vi "TruPlasma3001.vi"() -> ()   [LabVIEW 2015]
panel:
  in  "Pset":dbl=150.0
  in  "Iset":dbl=5000.0
  in  "Uset":dbl=800.0
  in  "Byte string":string
  out "Bytes recieved":u32
  out "Bytes sent":u32
  in  "Boolean":bool
  out "string":string
  in  "CMD_L":string="ÿ"
  in  "CMD_H":string="ÿ"
  in  "reference":refnum<visa-resource-name>
  out "error out":errorcluster
  out "Command recieved":string
  # "Mains Relays: (1)On (0)Off\nPower: Off(0), On(1)\nReset arc counters: 1\n-\nAnalog: (1)\nPC Controls TruPlasma(1), Monitoring only(0)\nProfibus control(1)\nDisplay control(1)"
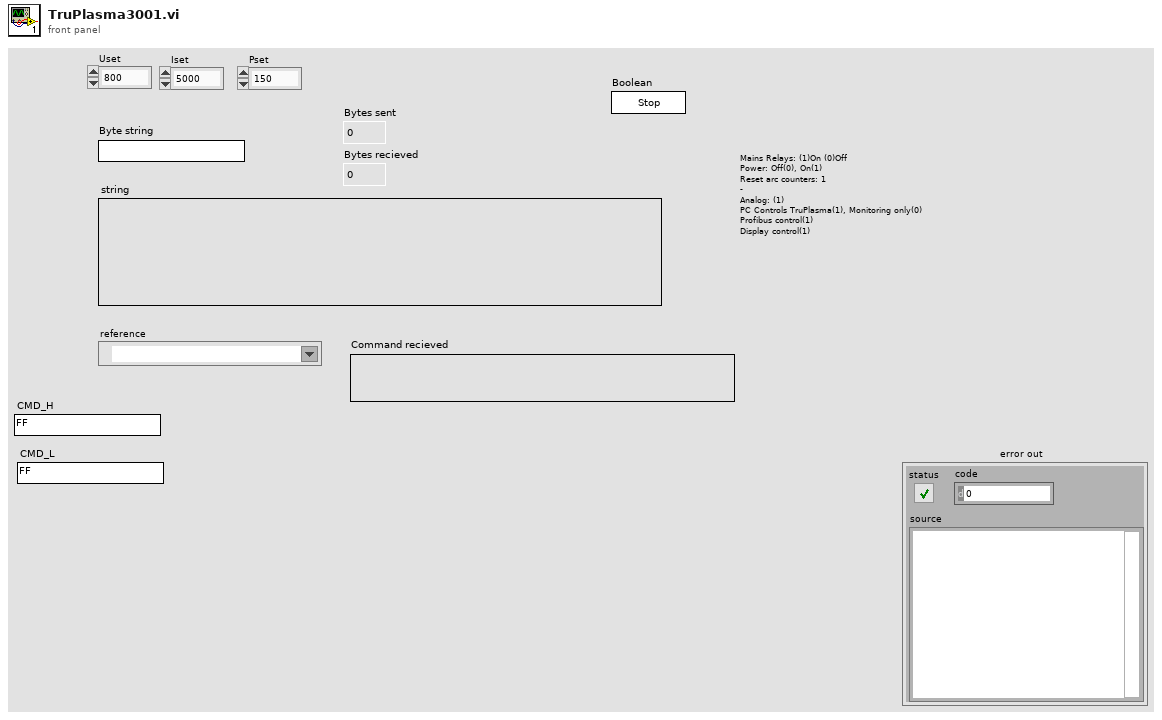
[diagram p1: front panel]
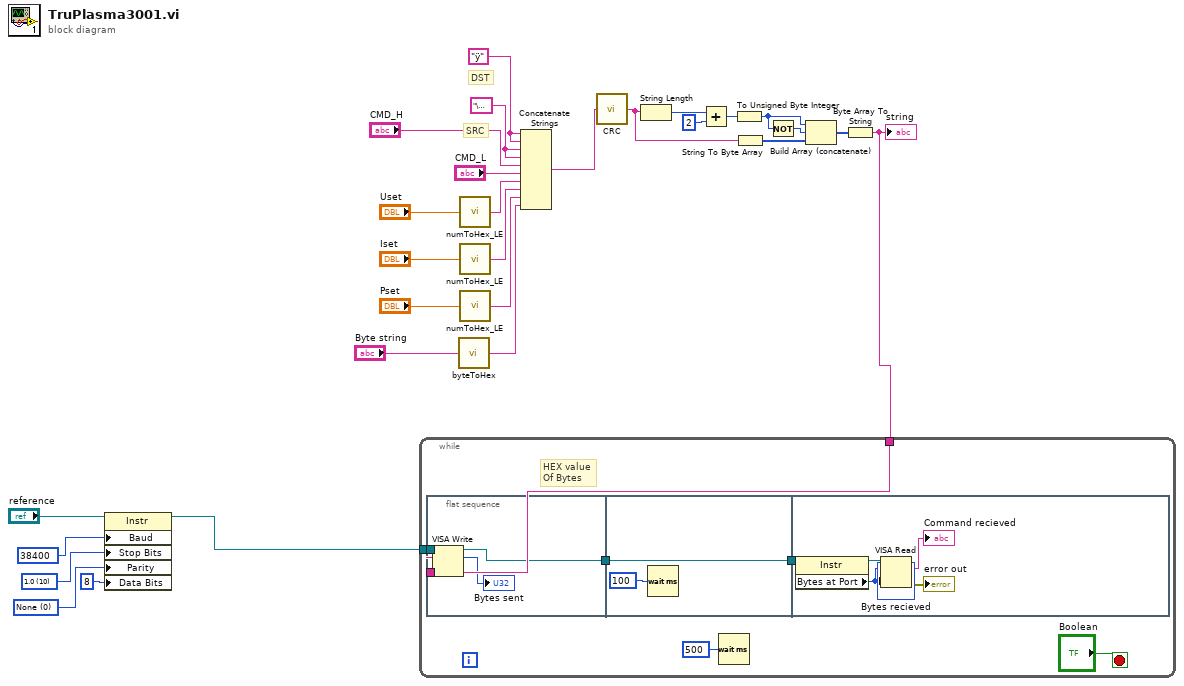
[diagram p0: block diagram]
diagram:
  w13 = u16 0 items=["None", "Odd", "Even", "Mark", "Space"] ("Serial Settings:Parity")
  w12 = u16 10 items=["1.0"=10, "1.5"=15, "2.0"=20] ("Serial Settings:Stop Bits")
  w27 = "\u0000" ("SRC")
  w28 = "ÿ" ("DST")
  # "SRC"
  # "DST"
  n1 = property class="Instr"(reference="reference", "Baud"=u32 38400 ("Serial Settings:Baud Rate"), "Stop Bits"=w12, "Parity"=w13, "Data Bits"=u16 8 ("Serial Settings:Data Bits")) -> (reference out=w9:refnum<visa-resource-name>)  [unwired: 1 in, 1 out]
  n2 = call "byteToHex.vi"("Byte string"="Byte string") -> ("HEX Value"=w3:string)
  n3 = call "numToHex_LE.vi"("Numeric"="Uset") -> ("string"=w6:string)
  n4 = call "numToHex_LE.vi"("Numeric"="Iset") -> ("string"=w5:string)
  n5 = call "numToHex_LE.vi"("Numeric"="Pset") -> ("string"=w4:string)
  n6 = Concatenate Strings(w28, w28, w27, w27, "CMD_H", "CMD_L", w6, w5, w4, w3) -> (w15:string)
  n7 = call "CRC.vi"("Input String"=w15) -> ("String w/ CRC"=w22:string)
  n8 = String Length(string=w22) -> (length=w24:i32)
  n9 = Add(x=w24, y=2) -> (x+y=w19:i32)
  n10 = To Unsigned Byte Integer(number=w19) -> (unsigned 8bit integer=w18:u8)
  n11 = String To Byte Array(string=w22) -> (unsigned byte array=w21:u8[])
  n12 = Not(x=w18) -> (.not. x?=w17:u8)
  n13 = Build Array (concatenate)(w18, w17, w21) -> (w20:u8[])
  n14 = Byte Array To String(unsigned byte array=w20) -> (string=w16:string)
  "string" <- w16
  n15 = while {
    tunnel: w16 -> [w32]
    tunnel: w9 -> [w30]
    stop <- "Boolean" stop-if-true
    # "HEX value\nOf Bytes"
    n16 = flat-sequence {
      tunnel: [w38] -> w34
      tunnel: w32 -> [w37]
      tunnel: w30 -> [w35]
      tunnel: w34 -> [w40]
      tunnel: [w40] -> w33
      tunnel: w33 -> [w41]
      frame #0 {
        n17 = VISA Write(VISA resource name=w35, write buffer=w37) -> (VISA resource name out=w38:refnum<visa-resource-name>, return count=→"Bytes sent":u32)  [unwired: 1 in, 1 out]
      }
      frame #1 {
        n18 = Wait (ms)(milliseconds to wait=u32 100) -> ()  [unwired: 1 out]
      }
      frame #2 {
        n19 = property class="Instr"(reference=w41) -> (reference out=w45:refnum<visa-resource-name>, "Bytes at Port"=w44:u32)  [unwired: 1 in, 1 out]
        "Bytes recieved" <- w44
        n20 = VISA Read(VISA resource name=w45, byte count=w44) -> (read buffer=→"Command recieved":string, error out=→"error out":errorcluster)  [unwired: 1 in, 2 out]
      }
    }
    n21 = Wait (ms)(milliseconds to wait=u32 500) -> ()  [unwired: 1 out]
  }
